vi "ADIS16470 Ref Get.vi"(8 "error in (no error)":errorcluster, 10 "refnum name":string="My IMU RefNum") -> (0 "error out":errorcluster, 3 "ADIS16470 Ref":T1={"DevStatus"={"status"=FALSE, "code"=0, "source"=""}, "Hardware Config"={"SPI Clock Rate (Hz)"=1000000.0, "IMU SPI Mode (3)"=enum."Mode 3 (Clk Idle High,Sample on Trailing)", "IMU Reset Pin"=enum."SPI Port CS2", "IMU SPI Bus"=enum."SPI On-Board, CS0", "IMU Data Ready Pin"=enum."SPI Port CS1"}, "End Calibration"=refnum, "Calibration Complete"=refnum, "Data FIFO"=refnum, "Status FIFO"=refnum, "Last Value Reference"=refnum, "Sychronous Process VI"=refnum, "Cmd FIFO"=refnum})   [LabVIEW 2018]
doc: "Gets the reference you specify. You first must set the reference with the RefNum Registry Set VI."
uses:
  Typedef/ADIS16470 Device Reference.ctl
  Typedef/ADIS16470 Hardware Configuration.ctl
  <vilib>/Rock Robotics/WPI/SPI/WPI_SPIMode.ctl
  <vilib>/Rock Robotics/SystemInterfaces/DIO/FPGA_DIOChannel.ctl
  <vilib>/Rock Robotics/SystemInterfaces/spilib/spi_bus.ctl
  Typedef/ADIS16470 Data.ctl
  Typedef/ADIS16470 Status.ctl
  Typedef/ADIS16470 Process.ctl
  Typedef/ADIS16470 Command Type.ctl
  <vilib>/Rock Robotics/WPI/Utilities/Refnum Registry Operation.ctl
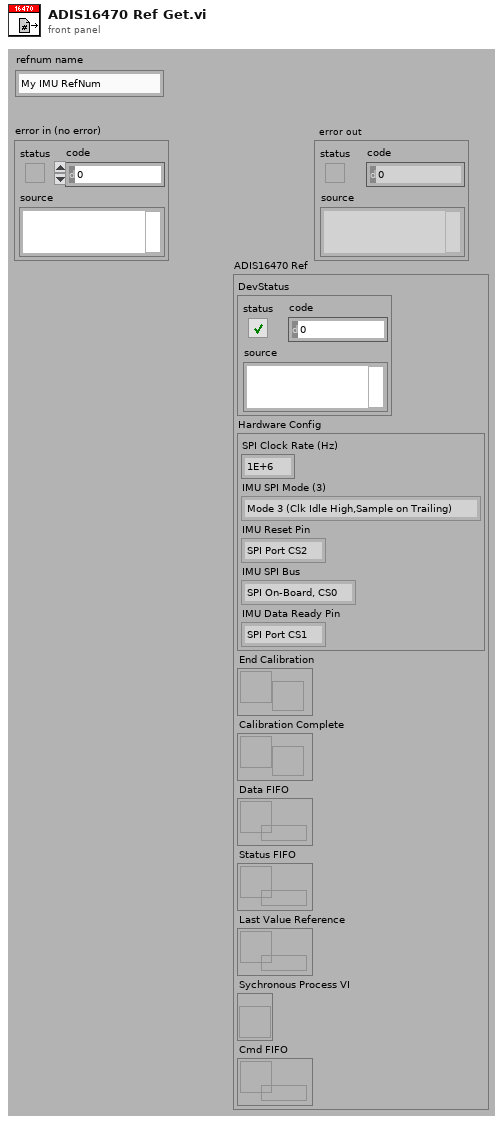
[diagram p1: front panel]
types:
  T1 = typedef "ADIS16470 Device Reference.ctl" = cluster{"DevStatus":errorcluster, "Hardware Config":T2, "End Calibration":refnum<notifier>, "Calibration Complete":refnum<notifier>, "Data FIFO":refnum<k33>, "Status FIFO":refnum<k33>, "Last Value Reference":refnum<data-value>, "Sychronous Process VI":T6, "Cmd FIFO":refnum<k33>}
  T2 = typedef "ADIS16470 Hardware Configuration.ctl" = cluster{"SPI Clock Rate (Hz)":dbl, "IMU SPI Mode (3)":T3, "IMU Reset Pin":T4, "IMU SPI Bus":T5, "IMU Data Ready Pin":T4}
  T3 = typedef "WPI_SPIMode.ctl" = enum16{"Mode 0 (Clk Idle Low,Sample on Leading)", "Mode 1 (Clk Idle Low,Sample on Trailing)", "Mode 2 (Clk Idle High,Sample on Leading)", "Mode 3 (Clk Idle High,Sample on Trailing)"}
  T4 = typedef "FPGA_DIOChannel.ctl" = enum8{"DIO 0", "DIO 1", "DIO 2", "DIO 3", "DIO 4", "DIO 5", "DIO 6", "DIO 7", "DIO 8", "DIO 9", "DIO MXP 0", "DIO MXP 1", "DIO MXP 2", "DIO MXP 3", "DIO MXP 4", "DIO MXP 5", "DIO MXP 6", "DIO MXP 7", "DIO MXP 8", "DIO MXP 9", "DIO MXP 10", "DIO MXP 11", "DIO MXP 12", "DIO MXP 13", "DIO MXP 14", "DIO MXP 15", "SPI Port CS1", "SPI Port CS2", "SPI Port CS3", "SPI Port MISO", "SPI Port MOSI", "Invalid"}
  T5 = typedef "spi_bus.ctl" = enum16{"SPI On-Board, CS0", "SPI On-Board, CS1", "SPI On-Board, CS2", "SPI On-Board, CS3", "SPI MXP", "Invalid"}
  T6 = typedef "ADIS16470 Process.ctl" = refnum<vi>
  T7 = typedef "Refnum Registry Operation.ctl" = enum16{"set", "get", "delete", "get all names", "read name"}
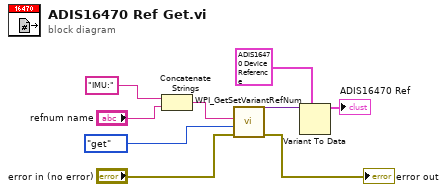
[diagram p0: block diagram]
diagram:
  n1 = Concatenate Strings("IMU:", "refnum name") -> (w4:string)
  n2 = call <vilib>:"WPI_GetSetVariantRefNum.vi"("error in (no error)"="error in (no error)", "Operation"=Refnum_Registry_Operation."get" ("menu"), "refnum name"=w4) -> ("error out"=→"error out":errorcluster, "DevRef"=w6:variant)  [unwired: 6 in, 1 out]
  n3 = Variant To Data(type=T1 {"DevStatus"={"status"=FALSE, "code"=0, "source"=""}, "Hardware Config"={"SPI Clock Rate (Hz)"=1000000.0, "IMU SPI Mode (3)"=enum."Mode 3 (Clk Idle High,Sample on Trailing)", "IMU Reset Pin"=enum."SPI Port CS2", "IMU SPI Bus"=enum."SPI On-Board, CS0", "IMU Data Ready Pin"=enum."SPI Port CS1"}, "End Calibration"=refnum, "Calibration Complete"=refnum, "Data FIFO"=refnum, "Status FIFO"=refnum, "Last Value Reference"=refnum, "Sychronous Process VI"=refnum, "Cmd FIFO"=refnum} ("ADIS16470DevRef"), Variant=w6) -> (data=→"ADIS16470 Ref":T1)  [unwired: 1 in, 1 out]
